vi "RoundCSG.vi"(5 "Decimal places":i8, 6 "Number":csg format="%#.10f") -> (2 "Rounded number":csg format="%#.10f")   [LabVIEW 2017, in "GPNumeric.lvlib"]
doc: "Rounds both the real and imaginary parts of the complex <B>Number</B> to a number of <B>Decimal places</B>.\n\nYou can set <B>Decimal places</B> to a negative number to round to nearest 10, nearest 100 and so on. E.g. to round 782-55i to the nearest hundred, you set <B>Decimal places</B> to -2 and the <B>Rounded number</B> will be 800-100i.\n\nThis VI is inlined.\n\n<B>Note</B> This VI uses the default IEEE 754 round-half-to-even rounding mode.\n\nSteen Schmidt\nGPower\n6/4 2014"
uses:
  GPNumeric.lvlib
panel:
  # "Copyright © 2014\nGPower\nSee enclosed license file for terms and conditions"
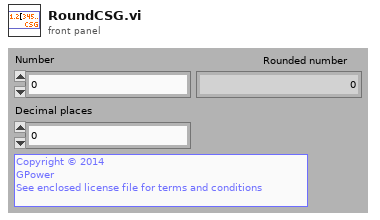
[diagram p1: front panel]
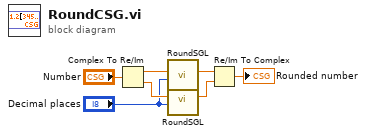
[diagram p0: block diagram]
diagram:
  n1 = Complex To Re/Im(x + iy="Number") -> (x=w6:sgl, y=w5:sgl)
  n2 = call "RoundSGL.vi"("Decimal places"="Decimal places", "Number"=w6) -> ("Rounded number"=w4:sgl)  [unwired: 5 in]
  n3 = call "RoundSGL.vi"("Decimal places"="Decimal places", "Number"=w5) -> ("Rounded number"=w3:sgl)  [unwired: 5 in]
  n4 = Re/Im To Complex(1:w3, 2:w4) -> (0:→"Rounded number":csg)
